vi "Open Adu Device By Serial Number.vi"(7 "Timeout":u32, 8 "error in (no error)":errorcluster, 11 "Serial Number":string) -> (0 "error out":errorcluster, 3 "function return":u32)   [LabVIEW 2015, in "AduHid.lvlib"]
doc: "void * __stdcall OpenAduDeviceBySerialNumber(const char* psSerialNumber,\n unsigned long iTimeout);"
uses:
  AduHid.lvlib
  AduHid.dll
  Windows/SysWOW64/kernel32.dll
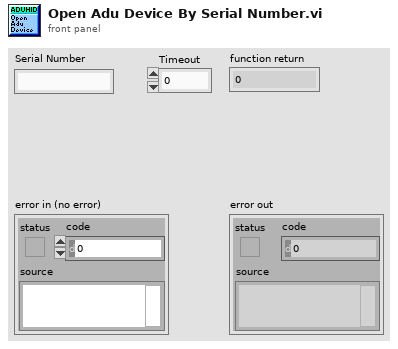
[diagram p1: front panel]
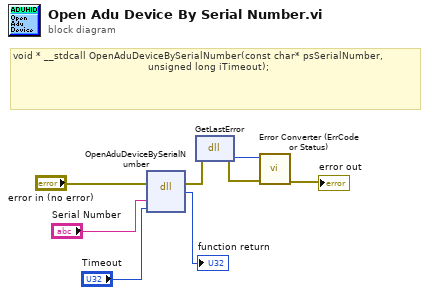
[diagram p0: block diagram]
diagram:
  # "void * __stdcall OpenAduDeviceBySerialNumber(const char* psSerialNumber,\n                                             unsigned long iTimeout);"
  n1 = dll-call lib="C:/Projects/CBTF Modules/Libraries/Ontrak ADU/API/AduHid.*" fn="OpenAduDeviceBySerialNumber"(error in="error in (no error)", "Serial Number"="Serial Number", "Timeout"="Timeout") -> (error out=w3:errorcluster, "return type"=→"function return":u32)  [unwired: 4 in, 1 out]
  n2 = dll-call lib="C:/Windows/SysWOW64/kernel32.dll" fn="GetLastError"(error in=w3) -> (error out=w2:errorcluster, "return type"=w1:u32)  [unwired: 2 in, 1 out]
  n3 = call "Error Converter (ErrCode or Status).vi"("error in (no error)"=w2, "error code"=w1) -> ("error out"=→"error out":errorcluster)  [unwired: 9 in]
